vi "get period.vi"(8 "error in":errorcluster, 11 "timing source in":refnum<class "absolute usec timing source.lvclass">) -> (0 "error out":errorcluster, 2 "period (ns)":i64, 3 "timing source out":refnum<class "absolute usec timing source.lvclass">)   [LabVIEW 2013, in "absolute usec timing source.lvclass"]
doc: "Returns the rate of the clock used by the selected timing source. This rate is the period measured in nanoseconds."
uses:
  absolute usec timing source.lvclass
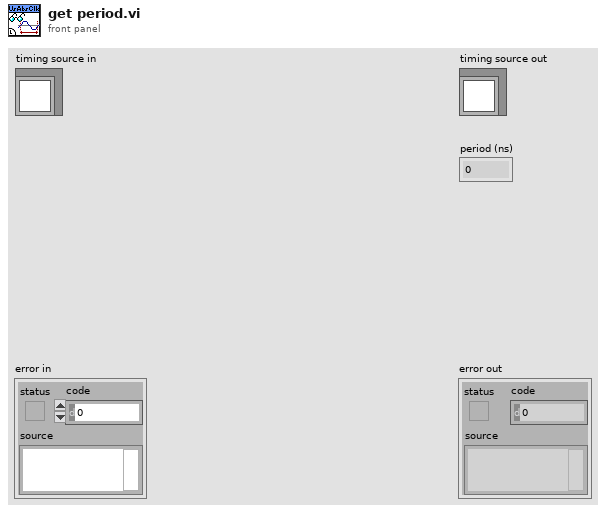
[diagram p1: front panel]
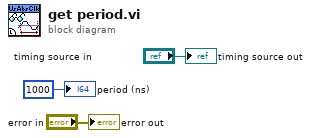
[diagram p0: block diagram]
diagram:
  "error out" <- "error in"
  "timing source out" <- "timing source in"
  "period (ns)" <- i64 1000 ("period (ns)")
